vi "Set Power.vi"(8 "error in (no error)":errorcluster, 11 "IMD in":refnum<class "IMD.lvclass">) -> (0 "error out":errorcluster, 1 "Parameter":cluster{"Name":string, "Value":string}, 2 "Last Power?":bool, 3 "IMD out":refnum<class "IMD.lvclass">)   [LabVIEW 2020, in "IMD.lvclass"]
uses:
  IMD.lvclass
  IMD.lvclass/IMD.ctl
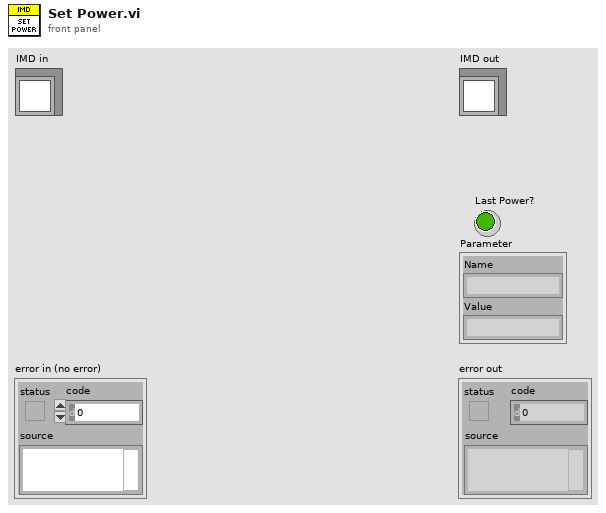
[diagram p1: front panel]
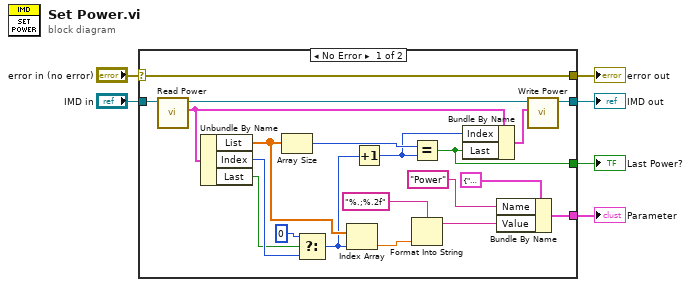
[diagram p0: block diagram]
diagram:
  n1 = case shown="No Error" "error in (no error)" {
    selector: "error in (no error)" -> [w7 w28]
    tunnel: [w7 w28] -> w5
    tunnel: [w8 w27] -> w3
    tunnel: "IMD in" -> [w10 w27]
    tunnel: [w16 _] -> w2
    tunnel: [w11 _] -> w1
    frame No Error {
      n2 = call "Read Power.vi"("IMD in"=w10) -> ("Power"=w25:cluster{"List":dbl[], "Index":i32, "Last":bool}, "IMD out"=w26:refnum<class "IMD.lvclass">)  [unwired: 9 in]
      n3 = Unbundle By Name(w25) -> ("List"=w20:dbl[], "Index"=w23:i32, "Last"=w21:bool)
      n4 = Array Size(array=w20) -> (size(s)=w19:i32)
      n5 = Select(t=0, s=w21, f=w23) -> (s? t:f=w18:i32)
      n6 = Index Array(array=w20, index=w18) -> (element=w9:dbl)
      n7 = Increment(x=w18) -> (x+1=w17:i32)
      n8 = Equal?(x=w19, y=w17) -> (x = y?=w16:bool)
      n9 = Format Into String(format string="%.;%.2f", w9) -> (resulting string=w12:string)  [unwired: 2 in, 1 out]
      n10 = Bundle By Name(cluster=w25, "Index"=w17, "Last"=w16) -> (w22:cluster{"List":dbl[], "Index":i32, "Last":bool})
      n11 = Bundle By Name(cluster=cluster{"Name":string, "Value":string} {"Name"="", "Value"=""} ("Change"), "Name"="Power", "Value"=w12) -> (w11:cluster{"Name":string, "Value":string})
      n12 = call "Write Power.vi"("Power"=w22, "IMD in"=w26) -> ("IMD out"=w8:refnum<class "IMD.lvclass">)  [unwired: 9 in]
    }
    frame Error {
    }
  }
  "error out" <- w5
  "IMD out" <- w3
  "Last Power?" <- w2
  "Parameter" <- w1
